vi "ReadDynamixelPosition.vi"(8 "error in (no error)":errorcluster, 9 "VISA resource name":refnum<visa-resource-name>, 10 "DynamixelPositions Queue":refnum<queue>, 11 "Notifier References":T1) -> (0 "error out":errorcluster, 3 "Dynamixel positions":dbl[](array[numeric]))   [LabVIEW 2013]
doc: "Reads Dynamixel torque off of the indicated Dynamixel and writes it to a queue.\n\nEric Schneider, March 2014"
uses:
  Data/TypeDefs/Notifiers.ctl
  Data/TypeDefs/UTM Location.ctl
  Data/TypeDefs/Sail Set Suggestions.ctl
  Data/TypeDefs/Rudder Set Suggestions.ctl
  Data/TypeDefs/OverrideInformation.ctl
  Data/TypeDefs/OverrideMode.ctl
  Data/TypeDefs/MotorSetup.ctl
  Data/TypeDefs/DynamixelSetupInfo.ctl
  Data/TypeDefs/AirmarStatus.ctl
  Data/TypeDefs/HardwareOnline.ctl
  Data/TypeDefs/DynamixelCycleTracker.ctl
  Data/TypeDefs/RC Input Values.ctl
  Classes/Waypoint/Waypoint.lvclass
  <instrlib>/Dynamixel Motor/Dynamixel Motor.lvlib
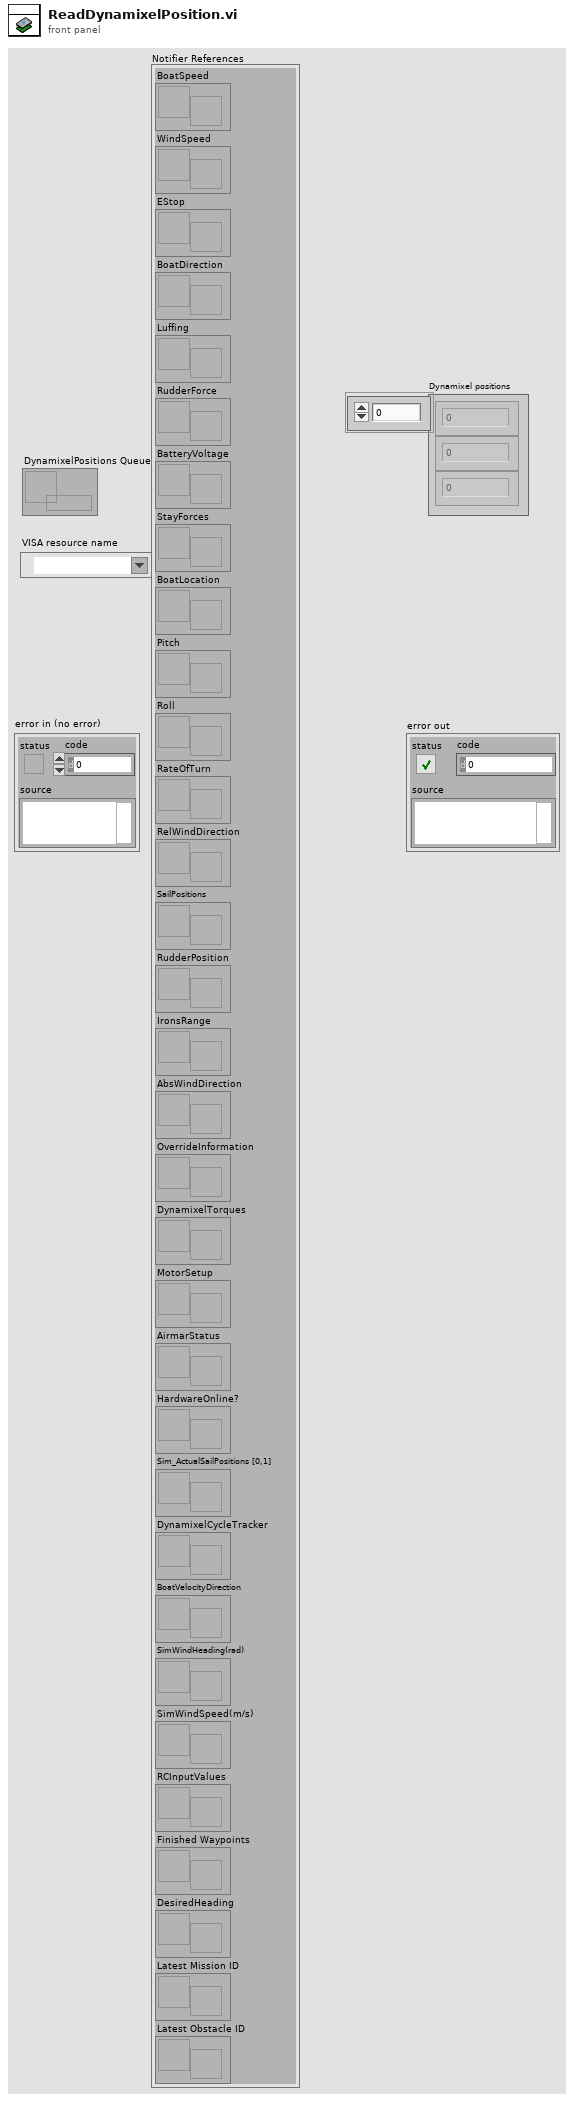
[diagram p1: front panel]
types:
  T1 = typedef "Notifiers.ctl" = cluster{"BoatSpeed":refnum<notifier>, "WindSpeed":refnum<notifier>, "EStop":refnum<notifier>, "BoatDirection":refnum<notifier>, "Luffing":refnum<notifier>, "RudderForce":refnum<notifier>, "BatteryVoltage":refnum<notifier>, "StayForces":refnum<notifier>, "BoatLocation":refnum<notifier>, "Pitch":refnum<notifier>, "Roll":refnum<notifier>, "RateOfTurn":refnum<notifier>, "RelWindDirection":refnum<notifier>, "SailPositions":refnum<notifier>, "RudderPosition":refnum<notifier>, "IronsRange":refnum<notifier>, "AbsWindDirection":refnum<notifier>, "OverrideInformation":refnum<notifier>, "DynamixelTorques":refnum<notifier>, "MotorSetup":refnum<notifier>, "AirmarStatus":refnum<notifier>, "HardwareOnline?":refnum<notifier>, "Sim_ActualSailPositions [0,1]":refnum<notifier>, "DynamixelCycleTracker":refnum<notifier>, "BoatVelocityDirection":refnum<notifier>, "SimWindHeading(rad)":refnum<notifier>, "SimWindSpeed(m/s)":refnum<notifier>, "RCInputValues":refnum<notifier>, "Finished Waypoints":refnum<notifier>, "DesiredHeading":refnum<notifier>, "Latest Mission ID":refnum<notifier>, "Latest Obstacle ID":refnum<notifier>}
  T2 = typedef "HardwareOnline.ctl" = cluster{"AirmarOnline":bool, "WindvaneOnline":bool, "HemisphereOnline":bool, "StayForceOnline":bool, "BatteryVoltageOnline":bool, "AccelerometerOnline":bool, "MainDynamixel Online":bool, "JibDynamixel Online":bool, "RudderDynamixel Online":bool}
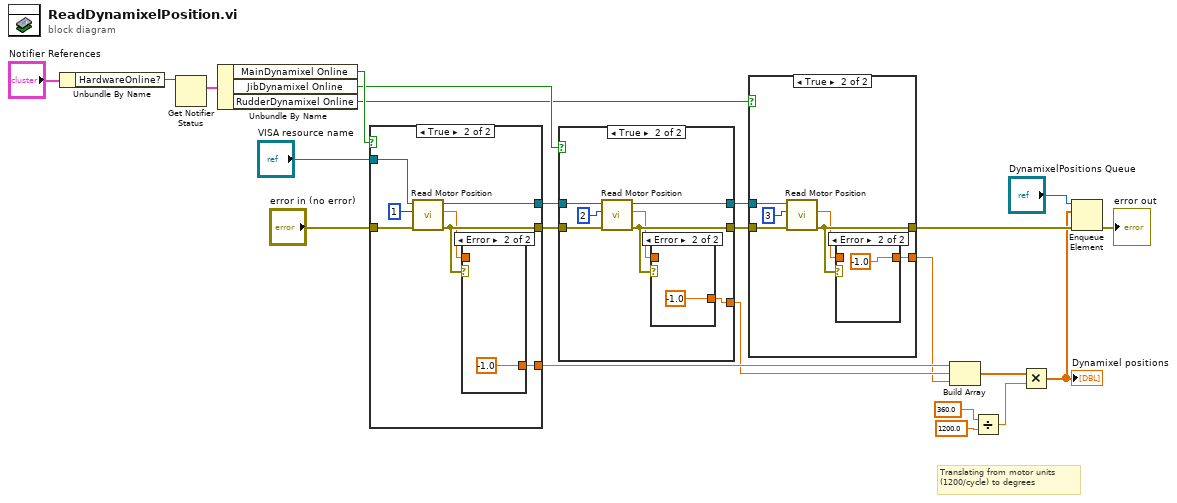
[diagram p0: block diagram]
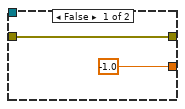
[diagram p2: hidden frame]
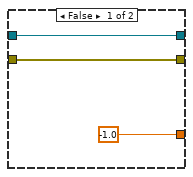
[diagram p4: hidden frame]
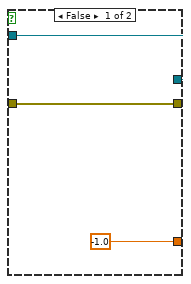
[diagram p6: hidden frame]
diagram:
  # "Translating from motor units (1200/cycle) to degrees"
  n1 = Unbundle By Name("Notifier References") -> ("HardwareOnline?"=w10:refnum<notifier>)
  n2 = Get Notifier Status(notifier=w10) -> (current notification=w9:T2)  [unwired: 1 in, 4 out]
  n3 = Unbundle By Name(w9) -> ("MainDynamixel Online"=w8:bool, "JibDynamixel Online"=w7:bool, "RudderDynamixel Online"=w6:bool)
  n4 = case shown="True" w8 {
    tunnel: "VISA resource name" -> [w25 w33]
    tunnel: "error in (no error)" -> [w24 w32]
    tunnel: [w25 w30] -> w20
    tunnel: [w24 w29] -> w19
    tunnel: [-1.0 ("Position (deg)") w27] -> w16
    frame False {
    }
    frame True {
      n5 = call <instrlib>:"Read Motor Position.vi"("error in (no error)"=w32, "Motor ID (0)"=u8 1, "VISA resource name"=w33) -> ("error out"=w29:errorcluster, "Position (deg)"=w28:dbl, "VISA resource name out"=w30:refnum<visa-resource-name>)  [unwired: 6 in]
      n6 = case shown="Error" w29 {
        tunnel: w28 -> [w34 _]
        tunnel: [w34 -1.0 ("Position (deg)")] -> w27
        frame No Error {
        }
        frame Error {
        }
      }
    }
  }
  n7 = case shown="True" w7 {
    tunnel: w20 -> [w36 w45]
    tunnel: w19 -> [w37 w44]
    tunnel: [w36 w43] -> w18
    tunnel: [w37 w41] -> w17
    tunnel: [-1.0 ("Position (deg)") w39] -> w15
    frame False {
    }
    frame True {
      n8 = call <instrlib>:"Read Motor Position.vi"("error in (no error)"=w44, "Motor ID (0)"=u8 2, "VISA resource name"=w45) -> ("error out"=w41:errorcluster, "Position (deg)"=w40:dbl, "VISA resource name out"=w43:refnum<visa-resource-name>)  [unwired: 6 in]
      n9 = case shown="Error" w41 {
        tunnel: w40 -> [w46 _]
        tunnel: [w46 -1.0 ("Position (deg)")] -> w39
        frame No Error {
        }
        frame Error {
        }
      }
    }
  }
  n10 = case shown="True" w6 {
    tunnel: w18 -> [_ w55]
    tunnel: w17 -> [w48 w54]
    tunnel: [-1.0 ("Position (deg)") w50] -> w14
    tunnel: [w48 w52] -> w13
    frame False {
    }
    frame True {
      n11 = call <instrlib>:"Read Motor Position.vi"("error in (no error)"=w54, "Motor ID (0)"=u8 3, "VISA resource name"=w55) -> ("error out"=w52:errorcluster, "Position (deg)"=w51:dbl)  [unwired: 6 in, 1 out]
      n12 = case shown="Error" w52 {
        tunnel: [w56 -1.0 ("Position (deg)")] -> w50
        tunnel: w51 -> [w56 _]
        frame No Error {
        }
        frame Error {
        }
      }
    }
  }
  n13 = Build Array(w16, w15, w14) -> (w5:dbl[])
  n14 = Divide(x=360.0, y=1200.0) -> (x/y=w2:dbl)
  n15 = Multiply(x=w5, y=w2) -> (x*y=w1:dbl[])
  "Dynamixel positions" <- w1
  n16 = Enqueue Element(queue="DynamixelPositions Queue", element=w1, error in (no error)=w13) -> (error out=→"error out":errorcluster)  [unwired: 1 in, 2 out]
